vi "kdtreesub.vi"(7 "depth_max":i32=10, 8 "mom":i32, 9 "out":dbl[][](array[numeric]), 10 "depth":i32, 11 "in":dbl[][](array[numeric])) -> (1 "out 2":dbl[][](array[numeric]))   [LabVIEW 2012]
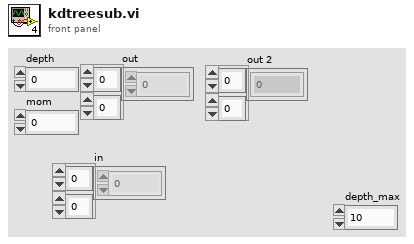
[diagram p1: front panel]
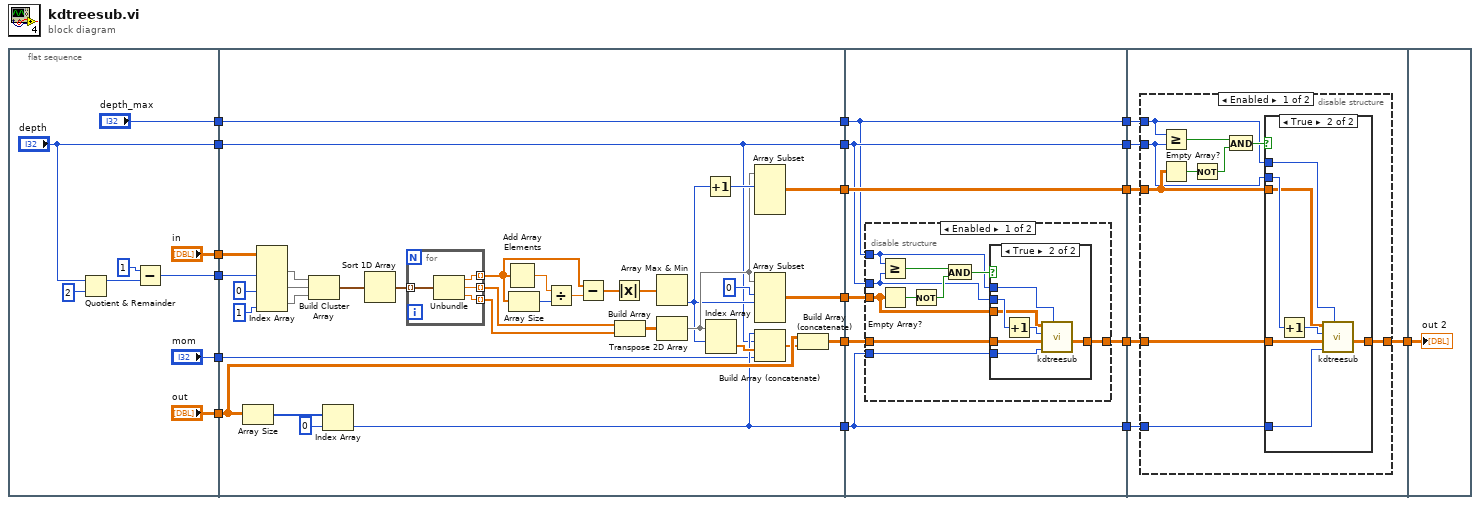
[diagram p0: block diagram]
diagram:
  n1 = flat-sequence {
    tunnel: ["out"] -> w15
    tunnel: ["depth"] -> w14
    tunnel: ["mom"] -> w9
    tunnel: [w21] -> w5
    tunnel: ["in"] -> w4
    tunnel: ["depth_max"] -> w2
    tunnel: [w40] -> w18
    tunnel: w15 -> [w39]
    tunnel: w14 -> [w32]
    tunnel: [w32] -> w13
    tunnel: [w38] -> w11
    tunnel: w9 -> [w37]
    tunnel: [w36] -> w8
    tunnel: [w35] -> w6
    tunnel: w5 -> [w34]
    tunnel: w4 -> [w33]
    tunnel: [w28] -> w3
    tunnel: w2 -> [w28]
    tunnel: w18 -> [w72]
    tunnel: [w71] -> w17
    tunnel: w13 -> [w67]
    tunnel: [w67] -> w12
    tunnel: w11 -> [w70]
    tunnel: [w70] -> w10
    tunnel: w8 -> [w69]
    tunnel: [w68] -> w7
    tunnel: w6 -> [w68]
    tunnel: w3 -> [w66]
    tunnel: [w66] -> w1
    tunnel: w17 -> [w97]
    tunnel: [w96] -> w16
    tunnel: w12 -> [w95]
    tunnel: w10 -> [w94]
    tunnel: w7 -> [w93]
    tunnel: w1 -> [w92]
    tunnel: w16 -> [w117]
    frame #0 {
      n2 = Quotient & Remainder(x="depth", y=2) -> (x-y*floor(x/y)=w26:i32)  [unwired: 1 out]
      n3 = Subtract(x=1 ("y"), y=w26) -> (x-y=w21:i32)
    }
    frame #1 {
      n4 = Array Size(array=w39) -> (size(s)=w31:i32[])
      n5 = Index Array(array=w33, index (col) #1=w34, index (col) #2=0 ("index (col)"), index (col) #3=1 ("index (col)")) -> (element #1=w55:dbl[], element #2=w54:dbl[], element #3=w53:dbl[])  [unwired: 3 in]
      n6 = Build Cluster Array(w55, w54, w53) -> (w52:cluster{dbl, dbl, dbl}[])
      n7 = Index Array(array=w31, index=0) -> (element=w38:i32)
      n8 = Sort 1D Array(array=w52) -> (sorted array=w51:cluster{dbl, dbl, dbl}[])
      n9 = for {
        tunnel: w51 -> [w65] mode=indexing
        tunnel: [w64] -> w50 mode=indexing
        tunnel: [w63] -> w48 mode=indexing
        tunnel: [w62] -> w47 mode=indexing
        n10 = Unbundle(w65) -> (w64:dbl, w63:dbl, w62:dbl)
      }
      n11 = Add Array Elements(numeric array=w50) -> (sum=w61:dbl)
      n12 = Array Size(array=w50) -> (size(s)=w60:i32)
      n13 = Divide(x=w61, y=w60) -> (x/y=w59:dbl)
      n14 = Subtract(x=w50, y=w59) -> (x-y=w58:dbl[])
      n15 = Absolute Value(x=w58) -> (abs(x)=w49:dbl[])
      n16 = Build Array(w48, w47) -> (w46:dbl[][])
      n17 = Array Max & Min(array=w49) -> (min index (indices)=w42:i32)  [unwired: 3 out]
      n18 = Transpose 2D Array(2D array=w46) -> (transposed array=w43:dbl[][])
      n19 = Increment(x=w42) -> (x+1=w44:i32)
      n20 = Index Array(array=w43, index (row)=w42) -> (element=w41:dbl[])  [unwired: 1 in]
      n21 = Array Subset(array=w43, index (row)=w44) -> (w35:dbl[][])  [unwired: 3 in]
      n22 = Array Subset(array=w43, index (row)=0 ("index"), length (row)=w42) -> (w36:dbl[][])  [unwired: 2 in]
      n23 = Build Array (concatenate)(w38, w32, w41, w37) -> (w29:dbl[])
      n24 = Build Array (concatenate)(w39, w29) -> (w40:dbl[][])
    }
    frame #2 {
      n25 = disable-structure shown="Enabled" {
        disable-tunnel: w72 -> [w82 w91]
        disable-tunnel: [w81 w91] -> w71
        disable-tunnel: w67 -> [w74 _]
        disable-tunnel: w70 -> [w80 _]
        disable-tunnel: w69 -> [w79 _]
        disable-tunnel: w66 -> [w73 _]
        frame Enabled {
          n26 = Greater Or Equal?(x=w73, y=w74) -> (x >= y?=w75:bool)
          n27 = Empty Array?(array=w79) -> (empty?=w78:bool)
          n28 = Not(x=w78) -> (.not. x?=w76:bool)
          n29 = And(x=w75, y=w76) -> (x .and. y?=w77:bool)
          n30 = case shown="True" w77 {
            tunnel: w82 -> [w83 w89]
            tunnel: [w83 w88] -> w81
            tunnel: w74 -> [_ w87]
            tunnel: w80 -> [_ w86]
            tunnel: w79 -> [_ w85]
            tunnel: w73 -> [_ w84]
            frame False {
            }
            frame True {
              n31 = Increment(x=w87) -> (x+1=w90:i32)
              n32 = call "kdtreesub.vi"("depth_max"=w84, "mom"=w86, "out"=w89, "depth"=w90, "in"=w85) -> ("out 2"=w88:dbl[][])  [unwired: 6 in]
            }
          }
        }
        frame Disabled {
        }
      }
    }
    frame #3 {
      n33 = disable-structure shown="Enabled" {
        disable-tunnel: w97 -> [w107 w116]
        disable-tunnel: [w106 w116] -> w96
        disable-tunnel: w95 -> [w102 _]
        disable-tunnel: w94 -> [w105 _]
        disable-tunnel: w93 -> [w104 _]
        disable-tunnel: w92 -> [w98 _]
        frame Enabled {
          n34 = Greater Or Equal?(x=w98, y=w102) -> (x >= y?=w103:bool)
          n35 = Empty Array?(array=w104) -> (empty?=w100:bool)
          n36 = Not(x=w100) -> (.not. x?=w99:bool)
          n37 = And(x=w103, y=w99) -> (x .and. y?=w101:bool)
          n38 = case shown="True" w101 {
            tunnel: w107 -> [w108 w114]
            tunnel: [w108 w113] -> w106
            tunnel: w102 -> [_ w112]
            tunnel: w105 -> [_ w111]
            tunnel: w104 -> [_ w110]
            tunnel: w98 -> [_ w109]
            frame False {
            }
            frame True {
              n39 = Increment(x=w112) -> (x+1=w115:i32)
              n40 = call "kdtreesub.vi"("depth_max"=w109, "mom"=w111, "out"=w114, "depth"=w115, "in"=w110) -> ("out 2"=w113:dbl[][])  [unwired: 6 in]
            }
          }
        }
        frame Disabled {
        }
      }
    }
    frame #4 {
      "out 2" <- w117
    }
  }
